vi "Did Interval Ellapse.vi"(1 "Future time coordinate (ms)":u32) -> (0 "Interval Ellapsed?":bool)   [LabVIEW 2021, in "Interval Timer.lvlib"]
uses:
  Interval Timer.lvlib
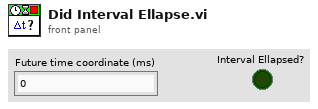
[diagram p1: front panel]
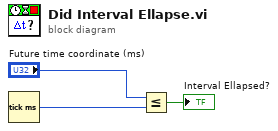
[diagram p0: block diagram]
diagram:
  n1 = Tick Count (ms)() -> (millisecond timer value=w2:u32)
  n2 = Less Or Equal?(x="Future time coordinate (ms)", y=w2) -> (x <= y?=→"Interval Ellapsed?":bool)
